vi "nobar.vi"(8 "error in (no error)":errorcluster, 10 "Horizontal Scrollbar Visibility":T1(ring), 11 "Pane in":refnum<vi>) -> (0 "error out":errorcluster, 3 "Pane ref out":refnum<vi>)   [LabVIEW 2015]
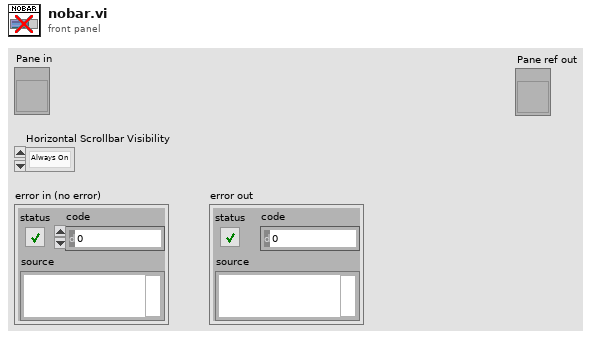
[diagram p1: front panel]
types:
  T1 = enum16{"Always On", "Always Off", "Off While Running"}
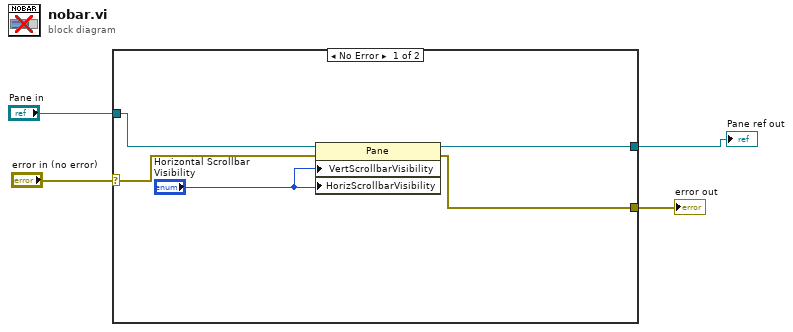
[diagram p0: block diagram]
diagram:
  n1 = case shown="No Error" "error in (no error)" {
    selector: "error in (no error)" -> [w6 w11]
    tunnel: "Pane in" -> [w8 w10]
    tunnel: [w7 w10] -> w2
    tunnel: [w5 w11] -> w1
    frame No Error {
      n2 = property on="Property Node" class="Pane"(reference=w8, error in=w6, "VertScrollbarVisibility"="Horizontal Scrollbar Visibility", "HorizScrollbarVisibility"="Horizontal Scrollbar Visibility") -> (reference out=w7:refnum<vi>, error out=w5:errorcluster)
    }
    frame Error {
    }
  }
  "error out" <- w1
  "Pane ref out" <- w2
